vi "TestManualJog.vi"() -> ()   [LabVIEW 2019]
uses:
  MotorController.lvclass
  enable_disable_enum_typedef.ctl
panel:
  in  "Serial Port":refnum<visa-resource-name>
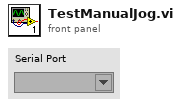
[diagram p1: front panel]
types:
  T1 = typedef "MotorController.lvclass/enable_disable_enum_typedef.ctl" = enum16{"Enable", "Disable"}
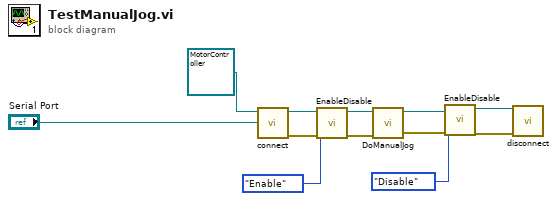
[diagram p0: block diagram]
diagram:
  n1 = call "connect.vi"("Serial Port"="Serial Port", "MotorController in"=refnum<class "MotorController.lvclass"> refnum) -> ("error out"=w5:errorcluster, "MotorController out"=w6:refnum<class "MotorController.lvclass">)  [unwired: 8 in]
  n2 = call "EnableDisable.vi"("error in (no error)"=w5, "Action"=enable_disable_enum_typedef."Enable", "MotorController in"=w6) -> ("error out"=w10:errorcluster, "MotorController out"=w9:refnum<class "MotorController.lvclass">)  [unwired: 7 in]
  n3 = call "DoManualJog.vi"("Error In"=w10, "MotorController in"=w9) -> ("Error Out"=w1:errorcluster, "MotorController out"=w4:refnum<class "MotorController.lvclass">)  [unwired: 8 in]
  n4 = call "EnableDisable.vi"("error in (no error)"=w1, "Action"=enable_disable_enum_typedef."Disable", "MotorController in"=w4) -> ("error out"=w2:errorcluster, "MotorController out"=w3:refnum<class "MotorController.lvclass">)  [unwired: 7 in]
  n5 = call "disconnect.vi"("error in (no error)"=w2, "MotorController in"=w3) -> ()  [unwired: 8 in, 2 out]
